vi "Write Data Raw.vi"(8 "error in (no error)":errorcluster, 10 "Data Raw":i32[][][][](array[numeric]), 11 "Experiment in":refnum<class "Experiment.lvclass">) -> (0 "error out":errorcluster, 3 "Experiment out":refnum<class "Experiment.lvclass">)   [LabVIEW 2019, in "Experiment.lvclass"]
uses:
  Experiment.lvclass
  Experiment.lvclass/Experiment.ctl
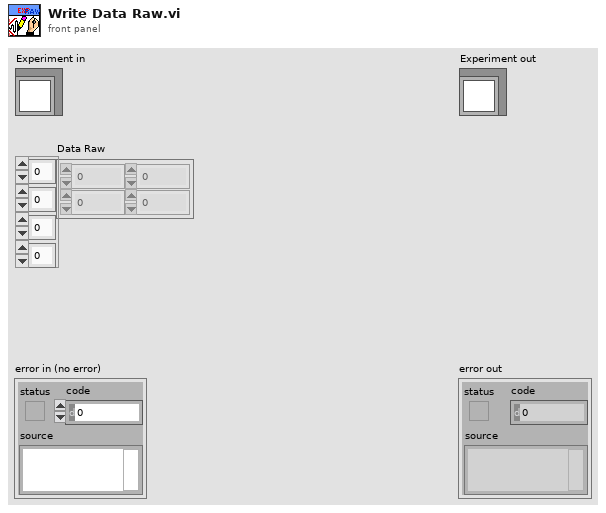
[diagram p1: front panel]
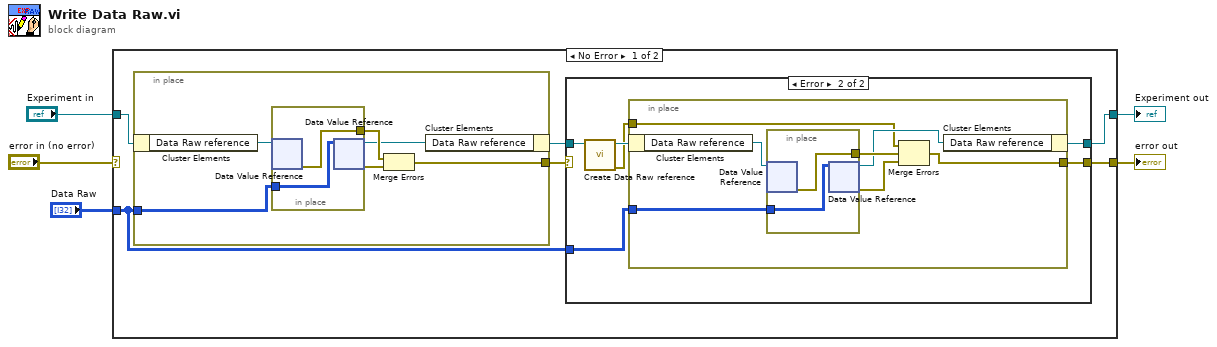
[diagram p0: block diagram]
diagram:
  n1 = case shown="No Error" "error in (no error)" {
    selector: "error in (no error)" -> [_ w38]
    tunnel: [w6 w38] -> w4
    tunnel: "Data Raw" -> [w9 _]
    tunnel: "Experiment in" -> [w10 w37]
    tunnel: [w8 w37] -> w1
    frame No Error {
      n2 = in-place {
        in-place-border: w9 -> [w32]
        in-place-border: [w29] -> w11
        n3 = in-place-cluster #1(w10) -> ("Data Raw reference"=w34:refnum<data-value>)
        n4 = in-place {
          in-place-border: w32 -> [w36]
          in-place-border: [w35] -> w31
          n5 = in-place-dvr #2(w34) -> (w35:errorcluster)  [unwired: 1 out]
          n6 = in-place-dvr #2(w36) -> (w30:refnum<data-value>, w33:errorcluster)
        }
        n7 = Merge Errors(w31, w33) -> (w29:errorcluster)
        n8 = in-place-cluster #1("Data Raw reference"=w30) -> (w7:refnum<class "Experiment.lvclass">)
      }
      n9 = case shown="Error" w11 {
        selector: w11 -> [w13 _]
        tunnel: [w13 w16] -> w6
        tunnel: w9 -> [_ w18]
        tunnel: [w12 w17] -> w8
        tunnel: w7 -> [w12 w15]
        frame No Error {
        }
        frame Error {
          n10 = call "Create Data Raw reference.vi"("Experiment in"=w15) -> ("error out"=w14:errorcluster, "Experiment out"=w19:refnum<class "Experiment.lvclass">)  [unwired: 9 in]
          n11 = in-place {
            in-place-border: [w22] -> w16
            in-place-border: w18 -> [w21]
            in-place-border: w14 -> [w20]
            n12 = in-place-cluster #3(w19) -> ("Data Raw reference"=w26:refnum<data-value>)
            n13 = in-place {
              in-place-border: [w28] -> w24
              in-place-border: w21 -> [w27]
              n14 = in-place-dvr #4(w26) -> (w28:errorcluster)  [unwired: 1 out]
              n15 = in-place-dvr #4(w27) -> (w23:refnum<data-value>, w25:errorcluster)
            }
            n16 = Merge Errors(w20, w24, w25) -> (w22:errorcluster)
            n17 = in-place-cluster #3("Data Raw reference"=w23) -> (w17:refnum<class "Experiment.lvclass">)
          }
        }
      }
    }
    frame Error {
    }
  }
  "error out" <- w4
  "Experiment out" <- w1
